vi "Task Type.vi"(11 "DataHandlerTask in":refnum<class "DataHandlerTask.lvclass">) -> (2 "Task Type":string)   [LabVIEW 2020, in "Volatus.lvlib" / "DataHandlerTask.lvclass"]
uses:
  DataHandlerTask.lvclass
  DataHandlerTask.lvclass/DataHandlerTask.ctl
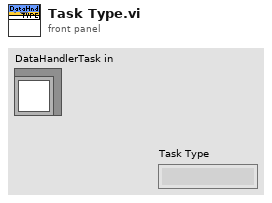
[diagram p1: front panel]
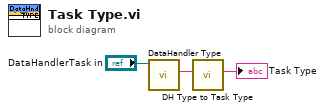
[diagram p0: block diagram]
diagram:
  n1 = call-dynamic "DataHandler Type.vi"("DataHandlerTask in"="DataHandlerTask in") -> ("DataHandler Type"=w2:string)  [unwired: 8 in, 2 out]
  n2 = call "DH Type to Task Type.vi"("DH Type"=w2) -> ("Task Type"=→"Task Type":string)  [unwired: 10 in]
